vi "Retrieve Actors.vi"(8 "error in (no error)":errorcluster, 11 "Target Store in":refnum<class "Target Store.lvclass">) -> (0 "error out":errorcluster, 1 "Actor Paths":path[](array[path]), 2 "Actors":string[](array[string]), 3 "Target Store out":refnum<class "Target Store.lvclass">)   [LabVIEW 2020, in "Add Actor.lvlib" / "Target Store.lvclass"]
uses:
  Target Store.lvclass
  MessageMakerProvider/AFPP Shared/Constants.vi
  MessageMakerProvider/AFPP Shared/AFPP Shared.lvlib
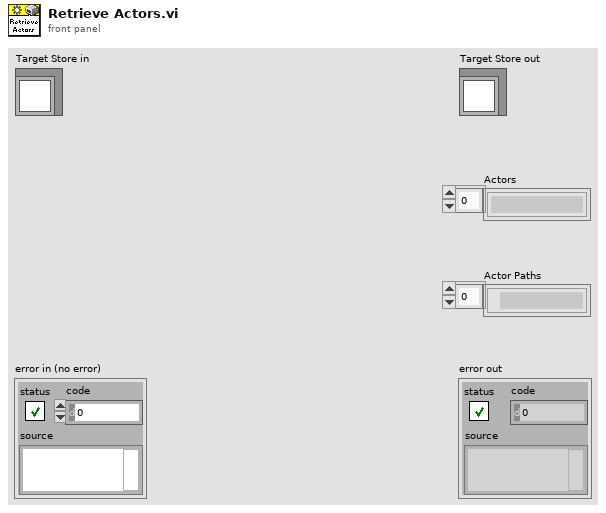
[diagram p1: front panel]
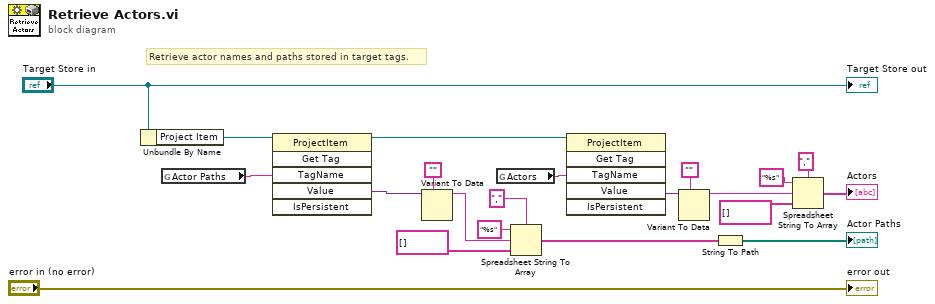
[diagram p0: block diagram]
diagram:
  # "Retrieve actor names and paths stored in target tags."
  n1 = Unbundle By Name("Target Store in") -> ("Project Item"=w17:refnum<vi>)
  n2 = global read "Constants.vi" "Actor Paths"() -> (w2:string)
  n3 = invoke class="ProjectItem" method="Get Tag"(reference=w17, "TagName"=w2) -> (reference out=w16:refnum<vi>, "Value"=w13:variant)  [unwired: 4 in, 4 out]
  n4 = Variant To Data(type="", Variant=w13) -> (data=w14:string)  [unwired: 1 in, 1 out]
  n5 = global read "Constants.vi" "Actors"() -> (w1:string)
  n6 = Spreadsheet String To Array(delimiter (Tab)=",", format string="%s", spreadsheet string=w14, array type (2D Dbl)=string[] [] ("Actors")) -> (array=w11:string[])
  n7 = invoke class="ProjectItem" method="Get Tag"(reference=w16, "TagName"=w1) -> ("Value"=w15:variant)  [unwired: 4 in, 5 out]
  n8 = Variant To Data(type="", Variant=w15) -> (data=w6:string)  [unwired: 1 in, 1 out]
  n9 = String To Path(string=w11) -> (path=→"Actor Paths":path[])
  n10 = Spreadsheet String To Array(delimiter (Tab)=",", format string="%s", spreadsheet string=w6, array type (2D Dbl)=string[] [] ("Actors")) -> (array=→"Actors":string[])
  "error out" <- "error in (no error)"
  "Target Store out" <- "Target Store in"
